vi "Distance2D.vi"(8 "y2":dbl, 9 "y1":dbl, 10 "x2":dbl, 11 "x1":dbl) -> (2 "distance":dbl)   [LabVIEW 2010, in "Waypoint.lvclass"]
uses:
  Waypoint.lvclass
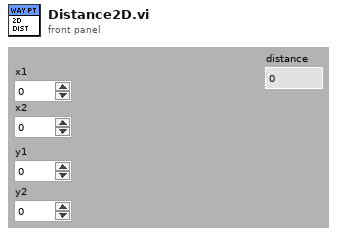
[diagram p1: front panel]
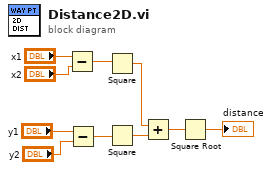
[diagram p0: block diagram]
diagram:
  n1 = Subtract(x="x1", y="x2") -> (x-y=w10:dbl)
  n2 = Subtract(x="y1", y="y2") -> (x-y=w9:dbl)
  n3 = Square(x=w10) -> (x^2=w7:dbl)
  n4 = Square(x=w9) -> (x^2=w8:dbl)
  n5 = Add(x=w7, y=w8) -> (x+y=w6:dbl)
  n6 = Square Root(x=w6) -> (sqrt(x)=→"distance":dbl)
